vi "Fake - 1 Session Unregistered.vi"(8 "error in":errorcluster) -> (0 "error out":errorcluster, 3 "session reservation out":refnum<class "Session Reservation.lvclass">)   [LabVIEW 2020, in "MeasurementServerTests.lvlib"]
uses:
  MeasurementServerTests.lvlib
  TestUtilities/TestUtilities.Runtime/Session Reservation Test Utilities/Session Reservation Test Utilities.lvlib
  Runtime/APIs/Session Management V1/Session Reservation/Session Reservation.lvclass
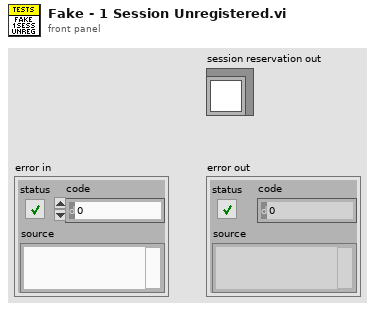
[diagram p1: front panel]
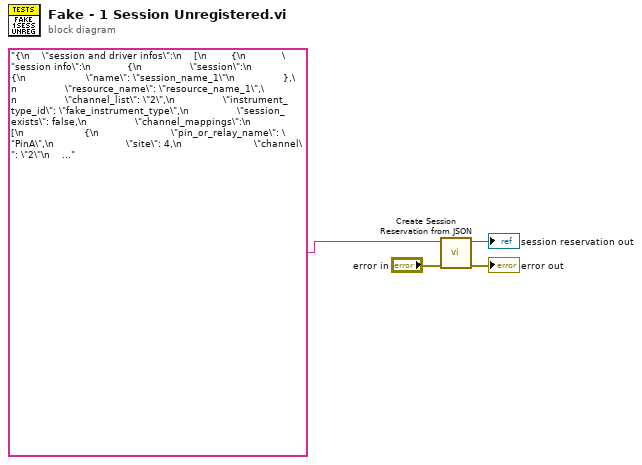
[diagram p0: block diagram]
diagram:
  n1 = call "Create Session Reservation from JSON.vi"("error in"="error in", "json"="{\n    \"session and driver infos\":\n    [\n        {\n            \"session info\":\n            {\n                \"session\":\n                {\n                    \"name\": \"session_name_1\"\n                },\n                \"resource_name\": \"resource_name_1\",\n                \"channel_list\": \"2\",\n                \"instrument_type_id\": \"fake_instrument_type\",\n                \"session_exists\": false,\n                \"channel_mappings\":\n                [\n                    {\n                        \"pin_or_relay_name\": \"PinA\",\n                        \"site\": 4,\n                        \"channel\": \"2\"\n                    }\n                ]\n            }\n        }\n    ],\n    \"dvr valid\": true\n}") -> ("error out"=→"error out":errorcluster, "session reservation out"=→"session reservation out":refnum<class "Session Reservation.lvclass">)  [unwired: 7 in, 1 out]
